vi "CutOffFilter.vi"(2 "Cutoff Radius":dbl=0.5 max=1.0 format="%.2f", 3 "Image In":T1 {"Dialogs" format="%.0b"}) -> (0 "FFT Out":T1 {"Dialogs" format="%.0b"}, 1 "Image Out":T1 {"Dialogs" format="%.0b"})   [LabVIEW 2024]
doc: "This VI zeros all frequencies outside a specified radius in the frequency domain. The cutoff ratio is expressed as a percentage of the maximum radius. It only works on greyscale images."
uses:
  <userlib>/ImageProcessing/QTLIB_2595_LV86/QT_Image.ctl
panel:
  # "This VI zeros all frequencies outside a specified radius in the frequency domain. The cutoff ratio is expressed as a percentage of the maximum radius. It only works on greyscale images."
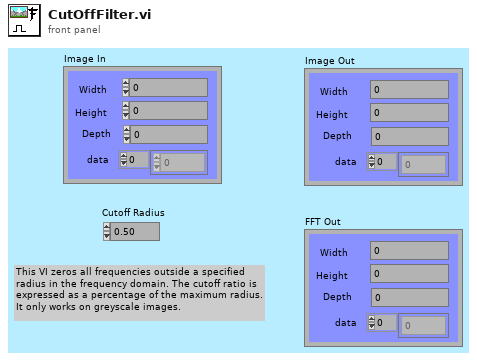
[diagram p1: front panel]
types:
  T1 = typedef "QT_Image.ctl" = cluster{"Width":i32, "Height":i32, "Depth":i32, "data":u8[], "Compressed data":u8[], "Color table":u32[], "Duration":i32, "Options":i32, "Timestamp":i32, "ID":i32, "Reserved":i32, "Dialogs":u32}
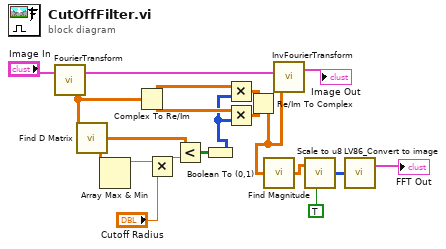
[diagram p0: block diagram]
diagram:
  n1 = call <userlib>:"FourierTransform.vi"("Image In"="Image In") -> ("Complex FT"=w1:cdb[][], "Image Out"=w19:T1)  [unwired: 1 in]
  n2 = call <userlib>:"Find D Matrix.vi"("Complex FT"=w1) -> ("Intensity Graph"=w2:dbl[][])
  n3 = Array Max & Min(array=w2) -> (max value=w11:dbl)  [unwired: 3 out]
  n4 = Complex To Re/Im(x + iy=w1) -> (x=w8:dbl[][], y=w7:dbl[][])
  n5 = Multiply(x=w11, y="Cutoff Radius") -> (x*y=w10:dbl)
  n6 = Less?(x=w2, y=w10) -> (x < y?=w13:bool[][])
  n7 = Boolean To (0,1)(Boolean=w13) -> (0, 1=w4:i16[][])
  n8 = Multiply(x=w8, y=w4) -> (x*y=w6:dbl[][])
  n9 = Multiply(x=w7, y=w4) -> (x*y=w5:dbl[][])
  n10 = Re/Im To Complex(1:w5, 2:w6) -> (0:w3:cdb[][])
  n11 = call <userlib>:"Find Magnitude.vi"("FFT {X}"=w3) -> ("Magnitude"=w15:dbl[][])
  n12 = call <userlib>:"InvFourierTransform.vi"("Complex matrix"=w3, "Image In"=w19) -> ("Image Out"=→"Image Out":T1)  [unwired: 1 in]
  n13 = call <userlib>:"Scale to u8.vi"("Log scaling?"=TRUE, "Intensity Graph"=w15) -> ("X"=w16:u8[][])
  n14 = call <userlib>:"LV86_Convert to image.vi"("Intensity Graph"=w16) -> ("Image Out"=→"FFT Out":T1)  [unwired: 2 in]
